vi "E4440A_PSA_Center_Span.vi"(8 "error in (no error)":errorcluster, 9 "Span (2 GHz)":dbl=2000000000.0, 10 "Center Frequency (2 GHz)":dbl=2000000000.0, 11 "VISA resource name":refnum<visa-resource-name>) -> (0 "error out":errorcluster, 3 "VISA resource name out":refnum<visa-resource-name>)   [LabVIEW 2015]
doc: "Configures the frequency range of the spectrum analyzer using the center frequency and the frequency span. If span corresponds to zero Hertz, then the spectrum analyzer operates in time-domain mode. Otherwise, spectrum analyzer operates in frequency-domain mode.\n\n Frequency Start = Center Frequency - Span/2\n Frequency Stop = Center Frequency + Span/2"
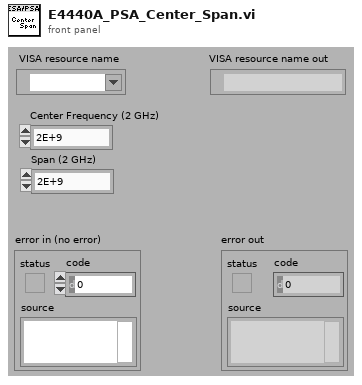
[diagram p1: front panel]
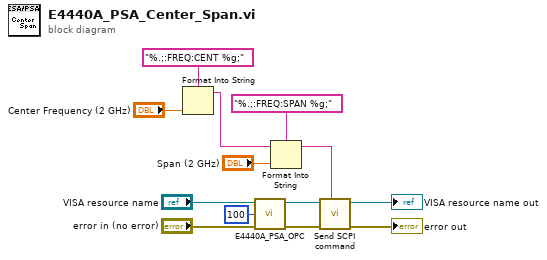
[diagram p0: block diagram]
diagram:
  n1 = Format Into String(format string="%.;:FREQ:CENT %g;", "Center Frequency (2 GHz)") -> (resulting string=w10:string)  [unwired: 2 in, 1 out]
  n2 = call "E4440A_PSA_OPC.vi"("error in (no error)"="error in (no error)", "Wait (1000ms)"=u32 100, "VISA resource name"="VISA resource name") -> ("error out"=w4:errorcluster, "VISA resource name out"=w2:refnum<visa-resource-name>)  [unwired: 7 in]
  n3 = Format Into String(format string="%.;:FREQ:SPAN %g;", initial string=w10, "Span (2 GHz)") -> (resulting string=w5:string)  [unwired: 1 in, 1 out]
  n4 = call "Send SCPI command.vi"("Send SCPI Command"=w5, "error in (no error)"=w4, "VISA resource name"=w2) -> ("error out"=→"error out":errorcluster, "VISA resource name out"=→"VISA resource name out":refnum<visa-resource-name>)  [unwired: 7 in]
